vi "仁科测控RS-KTC-N01空调控制器.vi"() -> ()   [LabVIEW 2016, in "环境动力监测库.lvlib" / "空调库.lvlib"]
uses:
  <vilib>/Utility/config.llb/NI_LVConfig.lvlib
panel:
  out "运行状态":T1
  out "传感器状态输出":T2
  out "温湿度解析":cluster{"温度":u16, "湿度":u16}
  out "告警状态":T3
  in  "解除告警":bool
  out "串口":string
  in  "查看型号":bool
  in  "重开串口":bool
  in  "设定参数":bool
  in  "遥控":bool
  out "通讯":bool
  # "A"
  # "A"
  # "℃"
  # "%"
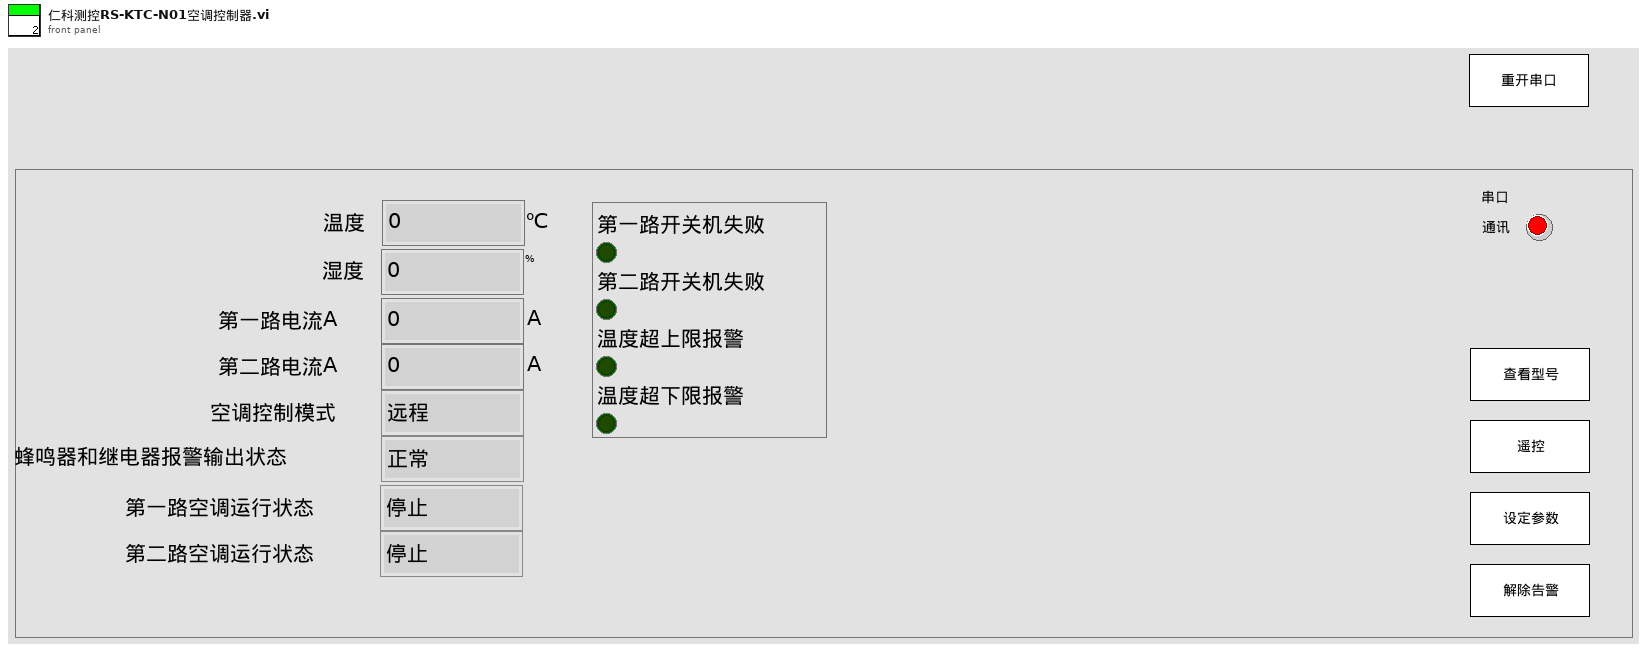
[diagram p1: front panel]
types:
  T1 = cluster{"第二路空调运行状态":enum16{"停止", "制冷", "制热", "未知"}, "第一路空调运行状态":enum16{"停止", "制冷", "制热", "未知"}}
  T2 = cluster{"第一路电流A":u16, "第二路电流A":u16, "空调控制模式":enum16{"远程", "自动"}, "蜂鸣器和继电器报警输出状态":enum16{"正常", "报警"}, "秒数高16位":u16, "秒数低16位":u16}
  T3 = cluster{"第一路开关机失败":bool, "第二路开关机失败":bool, "温度超上限报警":bool, "温度超下限报警":bool}
  T4 = enum32{"Bad", "Idle", "Run top level", "Running"}
  T5 = typedef "NI_LVConfig.lvlib/Config Data RefNum.ctl" = refnum<k1>
  T6 = cluster{"漏水监测输出":cluster{"漏水监测告警":bool, "告警内容":string}, "门禁监测输出":cluster{"门禁监测告警":bool, "告警内容":string}, "门禁监测输出2":cluster{"门禁监测告警":bool, "告警内容":string}, "温湿度监测输出":cluster{"温湿度监测告警":bool, "告警内容":string}, "烟雾监测输出":cluster{"烟雾监测告警":bool, "告警内容":string}, "空调监测输出":cluster{"空调监测告警":bool, "告警内容":string}, "自动重合闸输出":cluster{"自动重合闸告警":bool, "告警内容":string}, "红外入侵输出":cluster{"红外入侵告警":bool, "告警内容":string}, "振动输出":cluster{"振动告警":bool, "告警内容":string}, "UPS输出":cluster{"UPS告警":bool, "告警内容":string}, "蓄电池输出":cluster{"蓄电池告警":bool, "告警内容":string}, "蓄电池输出2":cluster{"蓄电池告警":bool, "告警内容":string}, "GPS输出":cluster{"定位告警":bool, "告警内容":string}, "北斗输出":cluster{"定位告警":bool, "告警内容":string}, "气象输出":cluster{"气象告警":bool, "告警内容":string}}
  T7 = cluster{"温湿度解析":cluster{"湿度":dbl, "温度":dbl}, "传感器状态输出":cluster{"第一路电流A":u16, "第二路电流A":u16, "空调控制模式":enum16{"远程", "自动"}, "蜂鸣器和继电器报警输出状态":enum16{"正常", "报警"}, "秒数高16位":u16, "秒数低16位":u16}, "告警状态":cluster{"第一路开关机失败":bool, "第二路开关机失败":bool, "温度超上限报警":bool, "温度超下限报警":bool}, "运行状态":cluster{"第一路空调运行状态":enum16{"停止", "制冷", "制热", "未知"}, "第二路空调运行状态":enum16{"停止", "制冷", "制热", "未知"}}}
  T8 = cluster{"第一路空调运行状态":enum16{"停止", "制冷", "制热", "未知"}, "第二路空调运行状态":enum16{"停止", "制冷", "制热", "未知"}}
  T9 = cluster{"温湿度":cluster{"状态":bool, "温度:":sgl, "湿度:":sgl, "详情  ":bool}, "空调":cluster{"状态":bool, "机柜温度:":sgl, "压缩机:":enum16{"停止", "运行"}, "电加热:":enum16{"停止", "运行"}, "详情  ":bool}, "排气扇":cluster{"排气扇:":enum16{"关闭", "打开"}, "详情  ":bool}, "冰箱":cluster{"冰箱:":enum16{"关闭", "打开"}, "详情  ":bool}}
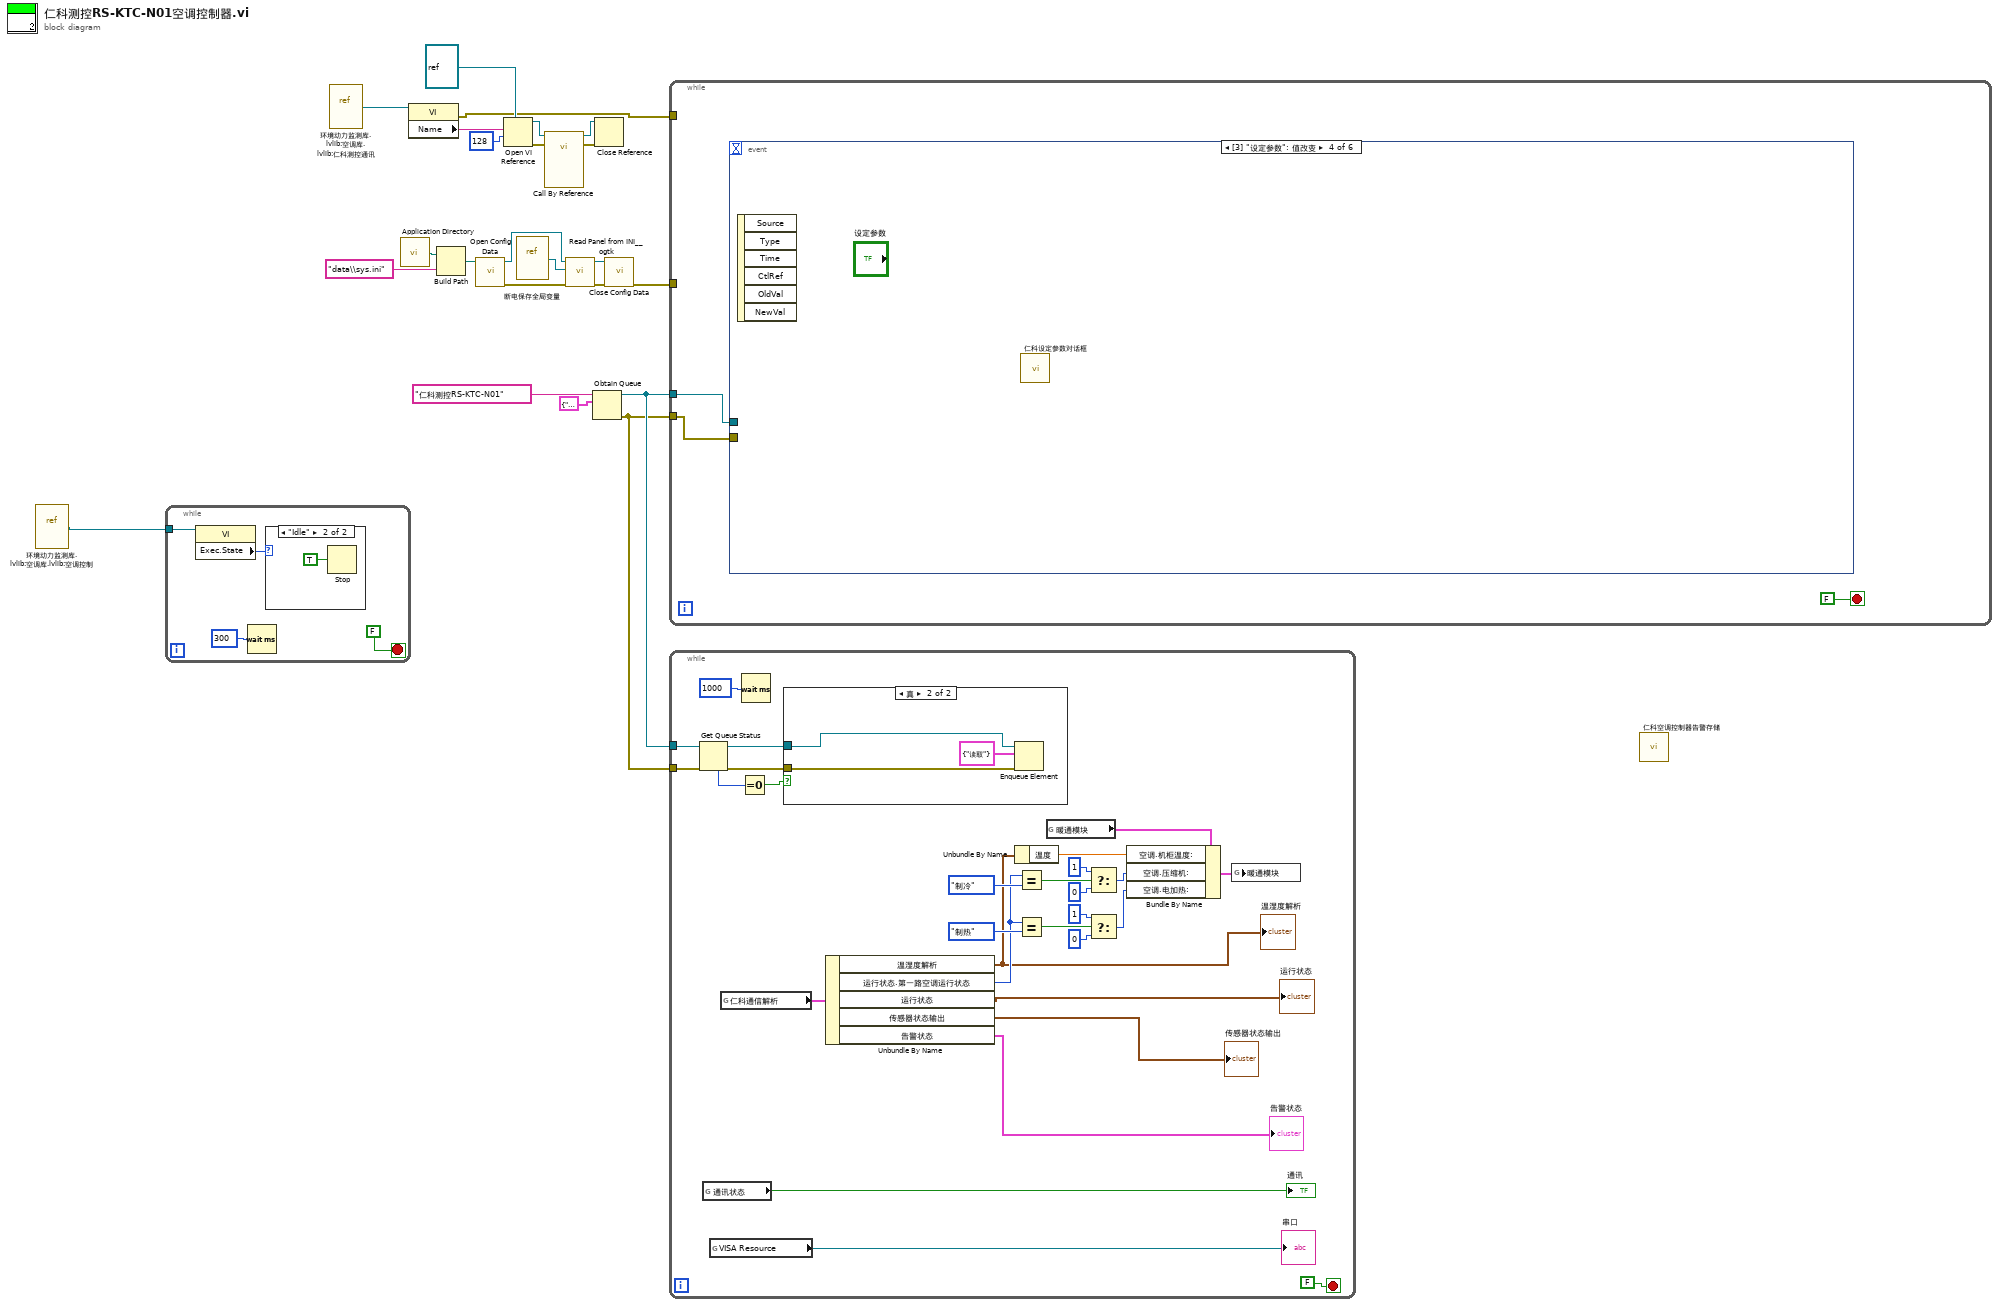
[diagram p0: block diagram]
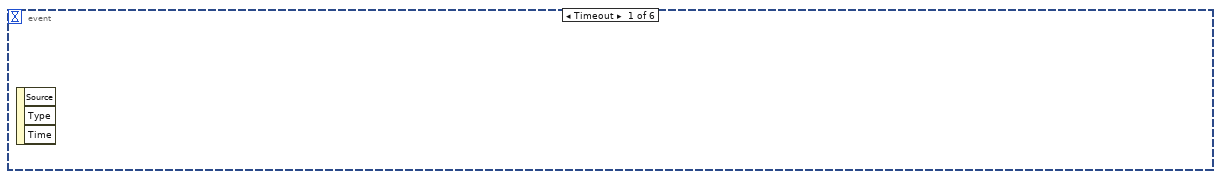
[diagram p4: hidden frame]
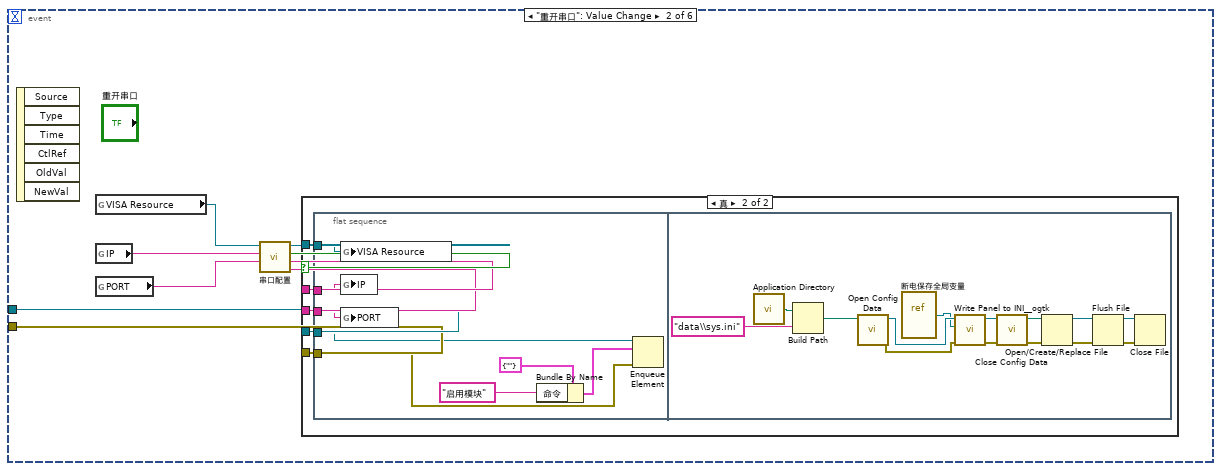
[diagram p5: hidden frame]
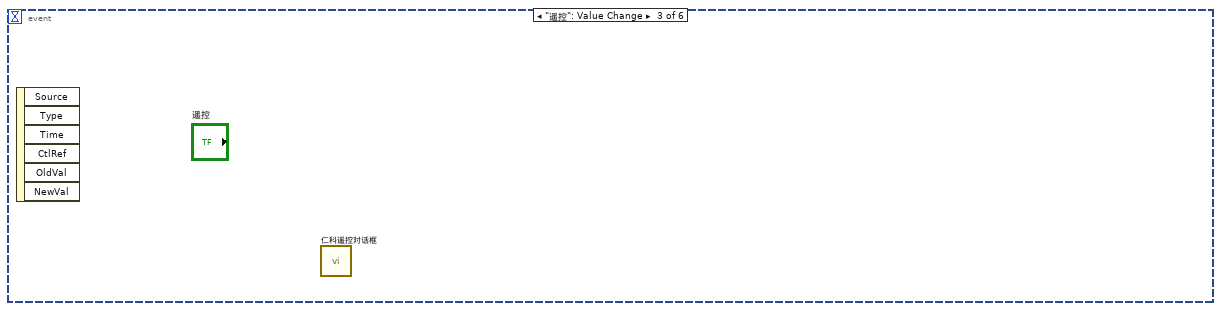
[diagram p7: hidden frame]
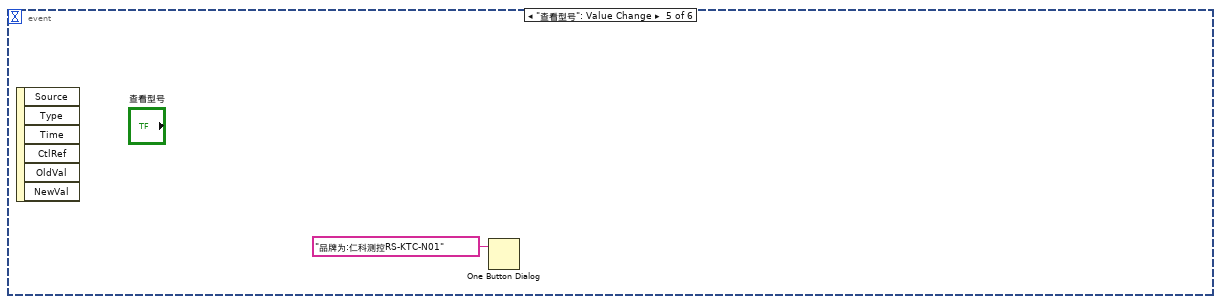
[diagram p8: hidden frame]
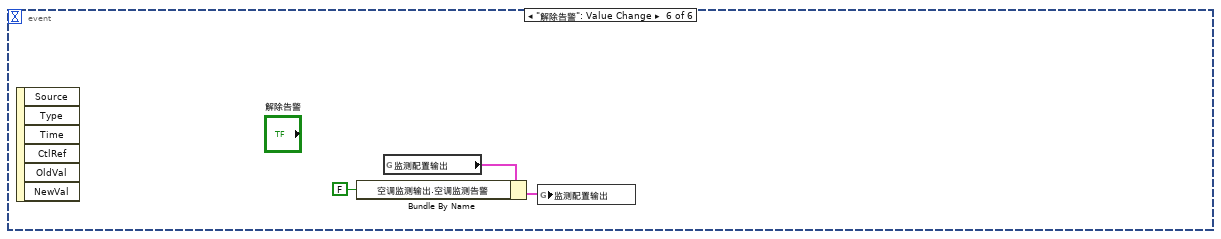
[diagram p9: hidden frame]
diagram:
  n1 = vi-ref "环境动力监测库.lvlib:空调库.lvlib:空调控制.vi"() -> (w1:refnum<vi>)
  n2 = while {
    tunnel: w1 -> [w27]
    stop <- FALSE stop-if-true
    n3 = property class="VI"(reference=w27) -> ("Exec.State"=w26:T4)  [unwired: 1 in, 2 out]
    n4 = Wait (ms)(milliseconds to wait=u32 300 ("等待时间（毫秒）")) -> ()  [unwired: 1 out]
    n5 = case shown="\"Idle\"" w26 {
      frame "Bad", Default {
      }
      frame "Idle" {
        n6 = Stop(stop? (T)=TRUE ("停止？(T)")) -> ()
      }
    }
  }
  n7 = vi-ref "环境动力监测库.lvlib:空调库.lvlib:仁科测控通讯.vi"() -> (w16:refnum<vi>)
  n8 = call <vilib>:"Application Directory.vi"() -> ("Application Directory"=w15:path)
  n9 = property class="VI"(reference=w16) -> (error out=w2:errorcluster, "Name"=w17:string)  [unwired: 1 in, 1 out]
  n10 = Build Path(base path=w15, name or relative path="data\\sys.ini" ("名称或相对路径")) -> (appended path=w13:path)
  n11 = call <vilib>:"Open Config Data.vi"("configuration file path"=w13) -> ("error out"=w9:errorcluster, "refnum"=w12:T5)  [unwired: 8 in, 1 out]
  n12 = Open VI Reference(type specifier VI Refnum (for type only)=refnum<vi> refnum, vi path=w17, options=128 ("选项")) -> (vi reference=w19:refnum<vi>, error out=w21:errorcluster)  [unwired: 3 in]
  n13 = vi-ref "断电保存全局变量.vi"() -> (w11:refnum<vi>)
  n14 = call-by-ref "?"(reference=w19, error in=w21) -> (reference out=w23:refnum<vi>, error out=w22:errorcluster)  [unwired: 12 in]
  n15 = call <userlib>:"Read Panel from INI__ogtk.vi"("error in (no error)"=w9, "VI ref"=w11, "refnum"=w12) -> ("error out"=w8:errorcluster, "refnum out"=w10:T5)  [unwired: 7 in]
  n16 = Obtain Queue(name (unnamed)="仁科测控RS-KTC-N01" ("名称（未命名）"), element data type=cluster{"命令":string} {"命令"="启用模块"} ("元素")) -> (queue out=w4:refnum<queue>, error out=w3:errorcluster)  [unwired: 3 in, 1 out]
  n17 = Close Reference(reference=w23, error in (no error)=w22) -> ()  [unwired: 1 out]
  n18 = call <vilib>:"Close Config Data.vi"("error in (no error)"=w8, "refnum"=w10) -> ("error out"=w7:errorcluster)  [unwired: 8 in, 1 out]
  n19 = while {
    tunnel: w7 -> [_]
    tunnel: w4 -> [w30]
    tunnel: w3 -> [w29]
    tunnel: w2 -> [_]
    stop <- FALSE stop-if-true
    n20 = event shown="[3] \"设定参数\": 值改变" {
      selector: _ -> [_ _ _ _ _ _]
      dyn-events: _ -> [_ _ _ _ _ _]
      timeout: _ -> [_ _ _ _ _ _]
      tunnel: w30 -> [_ w33 _ _ _ _]
      tunnel: w29 -> [_ w32 _ _ _ _]
      event Timeout {
        n21 = event-data() -> ()  [unwired: 1 in, 3 out]
      }
      event "重开串口": Value Change {
        n22 = event-data() -> ()  [unwired: 1 in, 6 out]
        n23 = global read "断电保存全局变量.vi" "VISA Resource"() -> (w40:refnum<visa-resource-name>)
        n24 = global read "断电保存全局变量.vi" "IP"() -> (w35:string)
        n25 = global read "断电保存全局变量.vi" "PORT"() -> (w34:string)
        n26 = call "串口配置.vi"("PORT"=w34, "IP"=w35, "请选择串口:"=w40) -> ("PORT 2"=w36:string, "IP 2"=w37:string, "确认 2"=w38:bool, "VISA资源名称 2"=w39:refnum<visa-resource-name>)  [unwired: 5 in]
        n27 = case shown="真" w38 {
          tunnel: w39 -> [_ w43]
          tunnel: w33 -> [_ w45]
          tunnel: w32 -> [_ w44]
          tunnel: w37 -> [_ w42]
          tunnel: w36 -> [_ w41]
          frame False {
          }
          frame True {
            n28 = flat-sequence {
              tunnel: w45 -> [w50]
              tunnel: w44 -> [w49]
              tunnel: w43 -> [w48]
              tunnel: w42 -> [w47]
              tunnel: w41 -> [w46]
              frame #0 {
                n29 = global write "断电保存全局变量.vi" "VISA Resource"(w48) -> ()
                n30 = global write "断电保存全局变量.vi" "IP"(w47) -> ()
                n31 = global write "断电保存全局变量.vi" "PORT"(w46) -> ()
                n32 = Bundle By Name(cluster=cluster{"命令":string} {"命令"=""} ("元素"), "命令"="启用模块" ("名称（未命名）")) -> (w51:cluster{"命令":string})
                n33 = Enqueue Element(queue=w50, element=w51, error in (no error)=w49) -> ()  [unwired: 1 in, 3 out]
              }
              frame #1 {
                n34 = call <vilib>:"Application Directory.vi"() -> ("Application Directory"=w66:path)
                n35 = Build Path(base path=w66, name or relative path="data\\sys.ini" ("名称或相对路径")) -> (appended path=w65:path)
                n36 = call <vilib>:"Open Config Data.vi"("configuration file path"=w65) -> ("error out"=w61:errorcluster, "refnum"=w64:T5)  [unwired: 8 in, 1 out]
                n37 = vi-ref "断电保存全局变量.vi"() -> (w63:refnum<vi>)
                n38 = call <userlib>:"Write Panel to INI__ogtk.vi"("error in (no error)"=w61, "VI ref"=w63, "refnum"=w64) -> ("error out"=w60:errorcluster, "refnum out"=w62:T5)  [unwired: 7 in]
                n39 = call <vilib>:"Close Config Data.vi"("error in (no error)"=w60, "refnum"=w62) -> ("error out"=w55:errorcluster, "file path"=w54:path)  [unwired: 8 in]
                n40 = Open/Create/Replace File(file path (use dialog)=w54, error in=w55) -> (refnum out=w58:refnum<file>, error out=w59:errorcluster)  [unwired: 4 in, 1 out]
                n41 = Flush File(refnum=w58, error in=w59) -> (refnum out=w57:refnum<file>, error out=w56:errorcluster)
                n42 = Close File(refnum=w57, error in=w56) -> ()  [unwired: 2 out]
              }
            }
          }
        }
      }
      event "遥控": Value Change {
        n43 = event-data() -> ()  [unwired: 1 in, 6 out]
        n44 = call "仁科遥控对话框.vi"() -> ()  [unwired: 12 in]
      }
      event "设定参数": Value Change {
        n45 = event-data() -> ()  [unwired: 1 in, 6 out]
        n46 = call "仁科设定参数对话框.vi"() -> ()  [unwired: 12 in]
      }
      event "查看型号": Value Change {
        n47 = event-data() -> ()  [unwired: 1 in, 6 out]
        n48 = One Button Dialog(message="品牌为:仁科测控RS-KTC-N01" ("消息")) -> ()  [unwired: 1 in, 1 out]
      }
      event "解除告警": Value Change {
        n49 = event-data() -> ()  [unwired: 1 in, 6 out]
        n50 = global read "断电保存全局变量.vi" "监测配置输出"() -> (w70:T6)
        n51 = Bundle By Name(cluster=w70, "空调监测输出.空调监测告警"=FALSE) -> (w71:T6)
        n52 = global write "断电保存全局变量.vi" "监测配置输出"(w71) -> ()
      }
    }
  }
  n53 = while {
    tunnel: w4 -> [w99]
    tunnel: w3 -> [w98]
    stop <- FALSE stop-if-true
    n54 = Get Queue Status(queue=w99, error in (no error)=w98) -> (queue out=w96:refnum<queue>, error out=w95:errorcluster, # elements in queue=w100:i32)  [unwired: 1 in, 5 out]
    n55 = global read "断电保存全局变量.vi" "通讯状态"() -> (→"通讯":bool)
    n56 = global read "断电保存全局变量.vi" "VISA Resource"() -> (→"串口":refnum<visa-resource-name>)
    n57 = global read "内部交互全局变量.vi" "仁科通信解析"() -> (w84:T7)
    n58 = Equal To 0?(x=w100) -> (x = 0?=w97:bool)
    n59 = Wait (ms)(milliseconds to wait=u32 1000 ("等待时间（毫秒）")) -> ()  [unwired: 1 out]
    n60 = case shown="真" w97 {
      tunnel: w96 -> [_ w103]
      tunnel: w95 -> [_ w102]
      frame False {
      }
      frame True {
        n61 = Enqueue Element(queue=w103, element=cluster{"命令":string} {"命令"="读取"} ("元素"), error in (no error)=w102) -> ()  [unwired: 1 in, 3 out]
      }
    }
    n62 = Unbundle By Name(w84) -> ("温湿度解析"=w74:cluster{"湿度":dbl, "温度":dbl}, "运行状态.第一路空调运行状态"=w80:enum16{"停止", "制冷", "制热", "未知"}, "运行状态"=→"运行状态":T8, "传感器状态输出"=→"传感器状态输出":T2, "告警状态"=→"告警状态":T3)
    "温湿度解析" <- w74
    n63 = Unbundle By Name(w74) -> ("温度"=w89:dbl)
    n64 = Equal?(x=w80, y=enum16{"停止", "制冷", "制热", "未知"}."制冷") -> (x = y?=w82:bool)
    n65 = Equal?(x=w80, y=enum16{"停止", "制冷", "制热", "未知"}."制热") -> (x = y?=w77:bool)
    n66 = global read "内部交互全局变量.vi" "暖通模块"() -> (w90:T9)
    n67 = Select(t=1, s=w82, f=0) -> (s? t:f=w85:i32)
    n68 = Select(t=1, s=w77, f=0) -> (s? t:f=w76:i32)
    n69 = Bundle By Name(cluster=w90, "空调.机柜温度:"=w89, "空调.压缩机:"=w85, "空调.电加热:"=w76) -> (w91:T9)
    n70 = global write "内部交互全局变量.vi" "暖通模块"(w91) -> ()
  }
  n71 = call "仁科空调控制器告警存储.vi"() -> ()  [unwired: 12 in]
